vi "checkAndCreateFolder.vi"(1 "storage path":path=path "C:/ni-rt/startup/datalog") -> (0 "dup path":path)   [LabVIEW 2021]
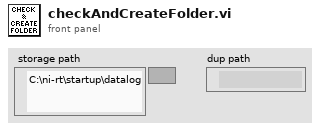
[diagram p1: front panel]
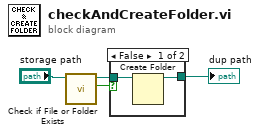
[diagram p0: block diagram]
diagram:
  n1 = call <vilib>:"Check if File or Folder Exists.vi"("path"="storage path") -> ("file or folder exists?"=w2:bool, "dup path"=w3:path)  [unwired: 1 in, 8 out]
  n2 = case shown="False" w2 {
    tunnel: w3 -> [w5 w7]
    tunnel: [w6 w7] -> w4
    frame False {
      n3 = Create Folder(path (use dialog)=w5) -> (created path=w6:path)  [unwired: 2 in, 2 out]
    }
    frame True {
    }
  }
  "dup path" <- w4
